vi "調整放大倍率.vi"() -> ()   [LabVIEW 2015]
uses:
  <vilib>/Utility/inputDevices.llb/mouseAcquire.vi
panel:
  out "放大倍率":sgl
  out "device ID":refnum<k1>
  out "Image":T1(plugin-control)
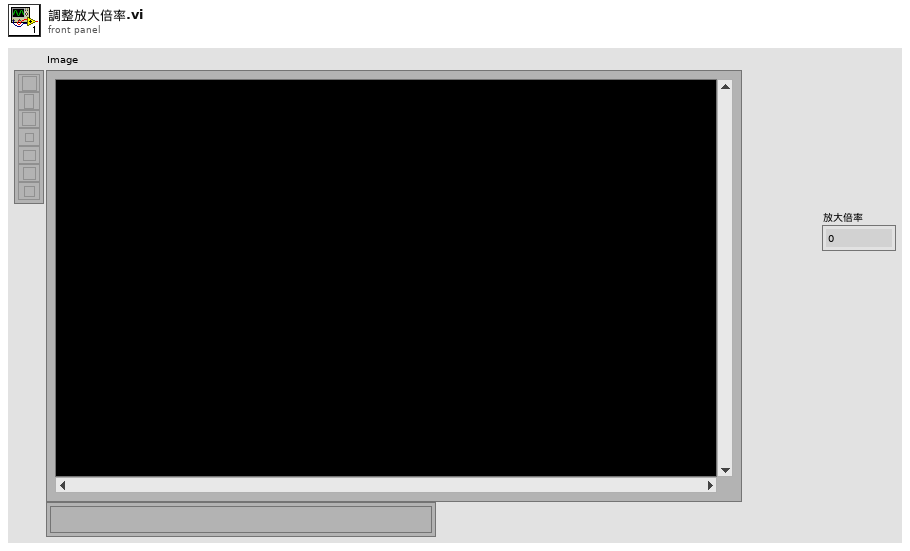
[diagram p1: front panel]
types:
  T1 = typedef "IMAQ Image.ctl" = refnum<image>
  T2 = enum16{"Always On", "Always Off", "Off While Running"}
  T3 = cluster{"Global Rectangle":i32[], "Contours":cluster{"Contour Type":u32, "ROI Type":u32, "Points":i32[]}[]}
  T4 = cluster{"Contour Type":u32, "ROI Type":u32, "Points":i32[]}[]
  T5 = cluster{"Contour Type":u32, "ROI Type":u32, "Points":i32[]}
  T6 = cluster{"Horizontal":i32, "Vertical":i32, "Scrolling":i32}
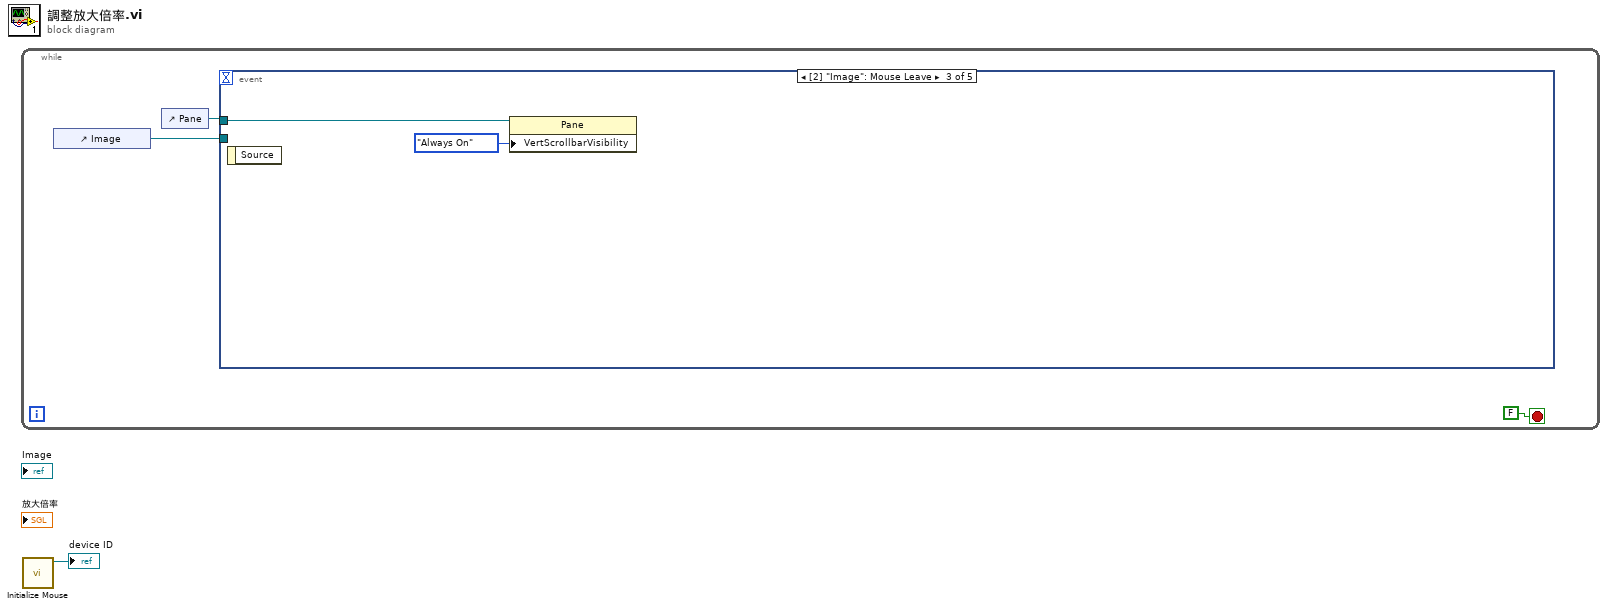
[diagram p0: block diagram]
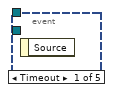
[diagram p2: hidden frame]
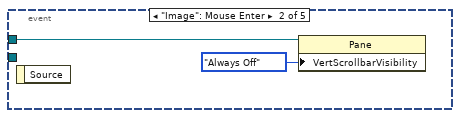
[diagram p3: hidden frame]
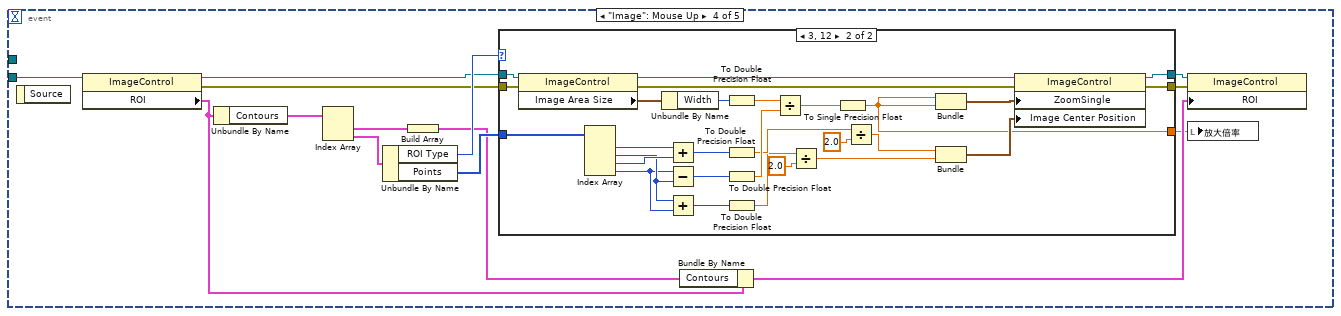
[diagram p4: hidden frame]
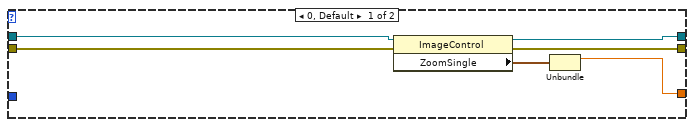
[diagram p5: hidden frame]
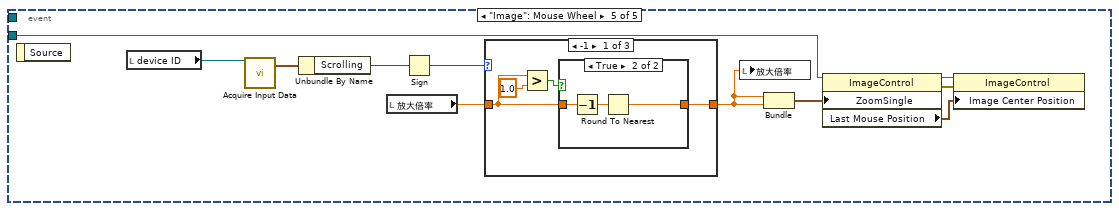
[diagram p6: hidden frame]
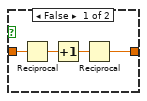
[diagram p7: hidden frame]
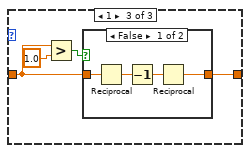
[diagram p9: hidden frame]
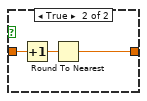
[diagram p10: hidden frame]
diagram:
  n1 = while {
    stop <- FALSE stop-if-true
    n2 = control-ref of="Image"() -> (w3:refnum<vi>)
    n3 = control-ref of="Pane"() -> (w2:refnum<vi>)
    n4 = event shown="[2] \"Image\": Mouse Leave" {
      selector: _ -> [_ _ _ _ _]
      dyn-events: _ -> [_ _ _ _ _]
      timeout: _ -> [_ _ _ _ _]
      tunnel: w3 -> [_ _ _ w10 w57]
      tunnel: w2 -> [_ w6 w8 _ _]
      event Timeout {
        n5 = event-data() -> ()  [unwired: 1 in, 1 out]
      }
      event "Image": Mouse Enter {
        n6 = event-data() -> ()  [unwired: 1 in, 1 out]
        n7 = property class="Pane"(reference=w6, "VertScrollbarVisibility"=T2."Always Off" ("Vertical Scrollbar Visibility")) -> ()  [unwired: 1 in, 2 out]
      }
      event "Image": Mouse Leave {
        n8 = event-data() -> ()  [unwired: 1 in, 1 out]
        n9 = property class="Pane"(reference=w8, "VertScrollbarVisibility"=T2."Always On" ("Vertical Scrollbar Visibility")) -> ()  [unwired: 1 in, 2 out]
      }
      event "Image": Mouse Up {
        n10 = event-data() -> ()  [unwired: 1 in, 1 out]
        n11 = property class="ImageControl"(reference=w10) -> (reference out=w14:refnum<vi>, error out=w12:errorcluster, "ROI"=w16:T3)  [unwired: 1 in]
        n12 = Unbundle By Name(w16) -> ("Contours"=w22:T4)
        n13 = Index Array(array=w22) -> (element #1=w18:T5, element #2=w21:T5)  [unwired: 2 in]
        n14 = Unbundle By Name(w21) -> ("ROI Type"=w20:u32, "Points"=w19:i32[])
        n15 = Build Array(w18) -> (w17:T4)
        n16 = case shown="3, 12" w20 {
          tunnel: w19 -> [_ w32]
          tunnel: w14 -> [w28 w56]
          tunnel: [w27 w36] -> w13
          tunnel: w12 -> [w25 w35]
          tunnel: [w24 w33] -> w11
          tunnel: [w23 w29] -> w9
          frame 0, Default {
            n17 = property class="ImageControl"(reference=w28, error in=w25) -> (reference out=w27:refnum<vi>, error out=w24:errorcluster, "ZoomSingle"=w26:cluster{"X":sgl, "Y":sgl})
            n18 = Unbundle(w26) -> ("X"=w23:sgl)  [unwired: 1 out]
          }
          frame 3, 12 {
            n19 = property class="ImageControl"(reference=w56, error in=w35) -> (reference out=w37:refnum<vi>, error out=w34:errorcluster, "Image Area Size"=w55:cluster{"Width":u32, "Height":u32})
            n20 = Index Array(array=w32) -> (element #1=w54:i32, element #2=w51:i32, element #3=w53:i32, element #4=w50:i32)  [unwired: 4 in]
            n21 = Unbundle By Name(w55) -> ("Width"=w45:u32)
            n22 = Add(x=w54, y=w53) -> (x+y=w42:i32)
            n23 = Subtract(x=w50, y=w51) -> (x-y=w47:i32)
            n24 = Add(x=w51, y=w50) -> (x+y=w40:i32)
            n25 = To Double Precision Float(number=w45) -> (double precision float=w44:dbl)
            n26 = To Double Precision Float(number=w42) -> (double precision float=w41:dbl)
            n27 = To Double Precision Float(number=w47) -> (double precision float=w46:dbl)
            n28 = To Double Precision Float(number=w40) -> (double precision float=w39:dbl)
            n29 = Divide(x=w44, y=w46) -> (x/y=w48:dbl)
            n30 = Divide(x=w39, y=2.0) -> (x/y=w30:dbl)
            n31 = To Single Precision Float(number=w48) -> (single precision float=w29:sgl)
            n32 = Divide(x=w41, y=2.0) -> (x/y=w31:dbl)
            n33 = Bundle(w29, w29) -> (w49:cluster{sgl, sgl})  [unwired: 1 in]
            n34 = Bundle(w31, w30) -> (w38:cluster{dbl, dbl})  [unwired: 1 in]
            n35 = property class="ImageControl"(reference=w37, error in=w34, "ZoomSingle"=w49, "Image Center Position"=w38) -> (reference out=w36:refnum<vi>, error out=w33:errorcluster)
          }
        }
        n36 = Bundle By Name(cluster=w16, "Contours"=w17) -> (w15:T3)
        n37 = property class="ImageControl"(reference=w13, error in=w11, "ROI"=w15) -> ()  [unwired: 2 out]
        n38 = local write "放大倍率"(w9) -> ()
      }
      event "Image": Mouse Wheel {
        n39 = event-data() -> ()  [unwired: 1 in, 1 out]
        n40 = local read "device ID"() -> (w67:refnum<k1>)
        n41 = call-poly <vilib>:"Acquire Input Data.vi"("device ID"=w67) -> ("axis info"=w66:T6)  [unwired: 15 in, 3 out]
        n42 = Unbundle By Name(w66) -> ("Scrolling"=w65:i32)
        n43 = local read "放大倍率"() -> (w63:sgl)
        n44 = Sign(1:w65) -> (0:w64:i32)
        n45 = case shown="-1" w64 {
          tunnel: w63 -> [w69 w79 w81]
          tunnel: [w68 w79 w80] -> w62
          frame -1 {
            n46 = Greater?(x=w69, y=1.0) -> (0:w70:bool)
            n47 = case shown="True" w70 {
              tunnel: w69 -> [w73 w78]
              tunnel: [w72 w76] -> w68
              frame False {
                n48 = Reciprocal(x=w73) -> (1/x=w74:sgl)
                n49 = Increment(x=w74) -> (x+1=w75:sgl)
                n50 = Reciprocal(x=w75) -> (1/x=w72:sgl)
              }
              frame True {
                n51 = Decrement(x=w78) -> (x-1=w77:sgl)
                n52 = Round To Nearest(number=w77) -> (nearest integer value=w76:sgl)
              }
            }
          }
          frame 0, Default {
          }
          frame 1 {
            n53 = Greater?(x=w81, y=1.0) -> (0:w82:bool)
            n54 = case shown="False" w82 {
              tunnel: w81 -> [w85 w90]
              tunnel: [w84 w88] -> w80
              frame False {
                n55 = Reciprocal(x=w85) -> (1/x=w86:sgl)
                n56 = Decrement(x=w86) -> (x-1=w87:sgl)
                n57 = Reciprocal(x=w87) -> (1/x=w84:sgl)
              }
              frame True {
                n58 = Increment(x=w90) -> (x+1=w89:sgl)
                n59 = Round To Nearest(number=w89) -> (nearest integer value=w88:sgl)
              }
            }
          }
        }
        n60 = local write "放大倍率"(w62) -> ()
        n61 = Bundle("放大倍率"=w62, "放大倍率"=w62) -> (w61:cluster{"放大倍率":sgl, "放大倍率":sgl})  [unwired: 1 in]
        n62 = property class="ImageControl"(reference=w57, "ZoomSingle"=w61) -> (reference out=w59:refnum<vi>, error out=w58:errorcluster, "Last Mouse Position"=w60:cluster{"X":i32, "Y":i32})  [unwired: 1 in]
        n63 = property class="ImageControl"(reference=w59, error in=w58, "Image Center Position"=w60) -> ()  [unwired: 2 out]
      }
    }
  }
  n64 = call <vilib>:"Initialize Mouse.vi"() -> ("device ID"=→"device ID":refnum<k1>)  [unwired: 10 in, 1 out]
